vi "GET_SupportData.vi"(8 "error in (no error)":errorcluster, 11 "FakedArray in":refnum<class "FakedArray.lvclass">) -> (0 "error out":errorcluster, 2 "Cluster":T1, 3 "FakedArray out":refnum<class "FakedArray.lvclass">)   [LabVIEW 2020, in "FakedArray.lvclass"]
uses:
  FakedArray.lvclass
  FakedArray.lvclass/FakedArray.ctl
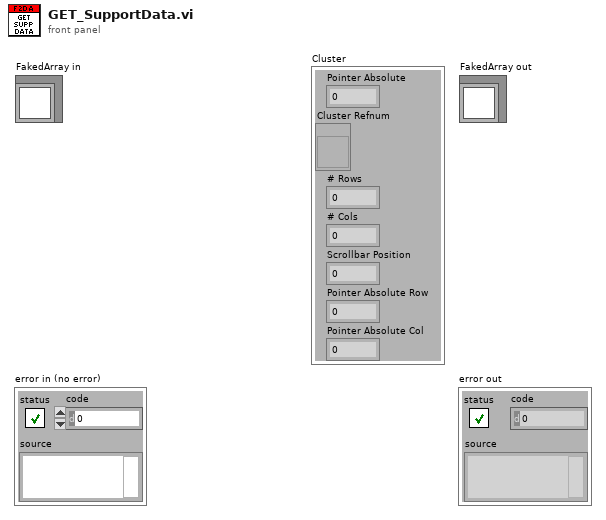
[diagram p1: front panel]
types:
  T1 = cluster{"Pointer Absolute":i32, "Cluster Refnum":refnum<vi>, "# Rows":i32, "# Cols":i32, "Scrollbar Position":i32, "Pointer Absolute Row":i32, "Pointer Absolute Col":i32}
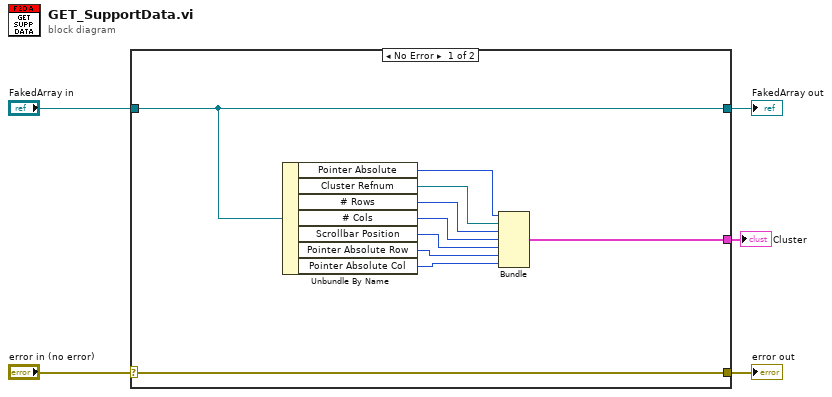
[diagram p0: block diagram]
diagram:
  n1 = case shown="No Error" "error in (no error)" {
    selector: "error in (no error)" -> [w15 w17]
    tunnel: [w15 w17] -> w4
    tunnel: [w14 w16] -> w2
    tunnel: "FakedArray in" -> [w14 w16]
    tunnel: [w6 _] -> w1
    frame No Error {
      n2 = Unbundle By Name(w14) -> ("Pointer Absolute"=w7:i32, "Cluster Refnum"=w8:refnum<vi>, "# Rows"=w9:i32, "# Cols"=w10:i32, "Scrollbar Position"=w11:i32, "Pointer Absolute Row"=w12:i32, "Pointer Absolute Col"=w13:i32)
      n3 = Bundle("Pointer Absolute"=w7, "Cluster Refnum"=w8, "# Rows"=w9, "# Cols"=w10, "Scrollbar Position"=w11, "Pointer Absolute Row"=w12, "Pointer Absolute Col"=w13) -> (w6:T1)  [unwired: 1 out]
    }
    frame Error {
    }
  }
  "error out" <- w4
  "FakedArray out" <- w2
  "Cluster" <- w1
